vi "VFRHA Volumetric Flow Rate of Humid Air (m3 to S).vi"(1 "Total Pressure of Humid Air":dbl[unit], 2 "Tceg":dbl[unit], 3 "MFRHA\nMass Flow Rate of Humid Air (Kg/s)":dbl[unit], 4 "RH":dbl) -> (0 "VFRHA":dbl[unit])   [LabVIEW 2018]
panel:
  out "VFRHA Volumetric Flow Rate of Humid Air\nVFRHA=MFRHA/DHA":dbl[unit](knob) scale=0.0..10.0
  out "Temprature Of Input Air\nKelvin Degree":dbl[unit](slide) scale=273.0..373.0
  out "Tk":dbl[unit]
  out "Temprature Of Input Air\nCentigrade Degree":dbl[unit](slide) scale=0.0..100.0
  out "Humidity of Input Air":dbl(knob) scale=0.0..100.0
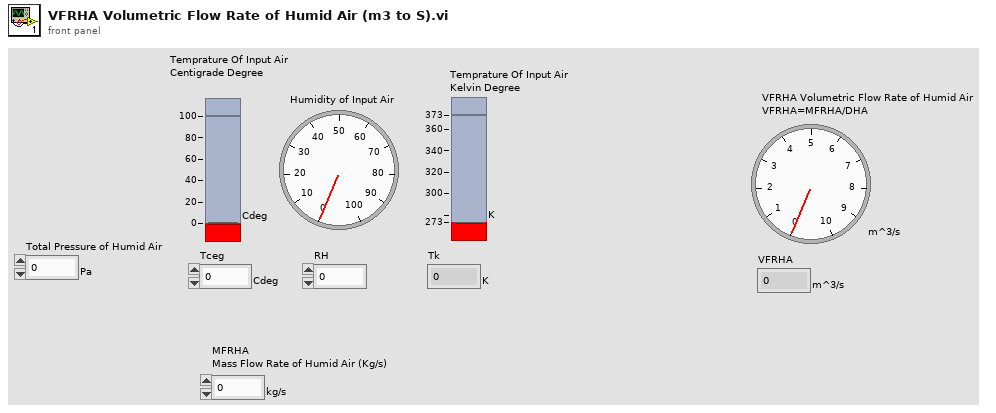
[diagram p1: front panel]
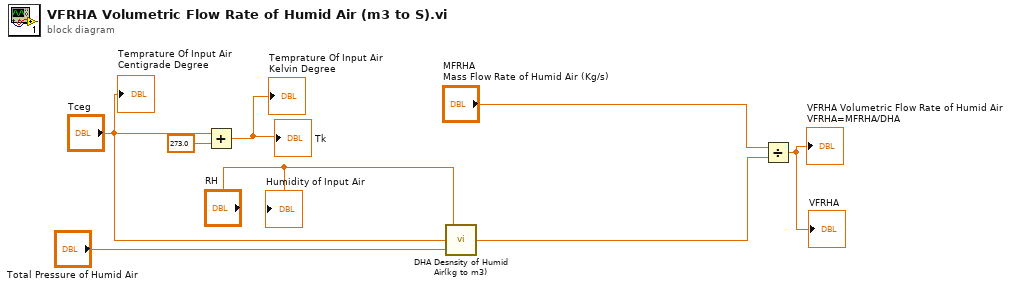
[diagram p0: block diagram]
diagram:
  n1 = Add(x="Tceg", y=dbl[unit] 273.0) -> (x+y=→"Tk" →"Temprature Of Input Air\nKelvin Degree":dbl[unit])
  n2 = call "DHA Desnsity of Humid Air(kg to m3).vi"("Total Pressure of Humid Air"="Total Pressure of Humid Air", "Tceg"="Tceg", "RH"="RH") -> ("DHA"=w4:dbl[unit])
  n3 = Divide(x="MFRHA\nMass Flow Rate of Humid Air (Kg/s)", y=w4) -> (x/y=→"VFRHA Volumetric Flow Rate of Humid Air\nVFRHA=MFRHA/DHA" →"VFRHA":dbl[unit])
  "Humidity of Input Air" <- "RH"
  "Temprature Of Input Air\nCentigrade Degree" <- "Tceg"
